vi "SLL DE Create DAQ INI File.vi"(8 "error in (no error)":errorcluster) -> (0 "error out":errorcluster)   [LabVIEW 2013]
doc: "Copyright © 2005, Soliton Technologies.\nAll rights reserved."
uses:
  Sub VIs/DAQ Engine/Controls/SLL DE List of Analog Outputs.ctl
  Sub VIs/DAQ Engine/Controls/SLL DE List of Digital Outputs.ctl
  Sub VIs/DAQ Engine/Controls/SLL DE DAQ Engine Parameters.ctl
  Sub VIs/DAQ Engine/Controls/SLL DE DAQ Parameters LV2Global Options.ctl
  Sub VIs/DAQ Engine/Controls/SLL DE List of Analog Inputs.ctl
  Sub VIs/DAQ Engine/Controls/SLL DE AO Min Max Range Checking Options.ctl
  Sub VIs/DAQ Engine/Controls/SLL DE List of AI Channel Type.ctl
panel:
  in  "DO Channel":T1=enum."STATION1_STOP TEST"
  in  "stop":bool
  in  "Tab Control":T2(tab)=enum."Page 11"
  in  "Stop":bool
  in  "Start":bool
  in  "Enable Acquisation and Control Types":T3={"Enable Analog Acqistation"=TRUE, "Enable Analog Control"=TRUE, "Enable Digital Acqistation"=TRUE, "Enable Digital Control"=TRUE}
  in  "OK 1":bool
  in  "DAQ Control Type":T4
  in  "OK 2":bool
  in  "DAQ Parameters":T5={"AI Sampling Rate (Samples/Sec)"=1000.0, "MvgAVG Window Size (# of Points)"=20, "Enable Filter"=TRUE, "Enable MvgAVG"=TRUE, "Circular Buffer Size (Sec)"=5.0, "AO Sampling Rate (Samples/Sec)"=1000.0, "Graph Update Rate (Samples/Sec)"=0.0, "File Logging Rate (Samples/Sec)"=500}
  in  "OK 3":bool
  in  "OK 4":bool
  in  "OK 5":bool
  in  "OK 6":bool
  in  "OK 7":bool
  in  "AO Safe Values":T7(array[cluster])
  in  "OK 8":bool
  in  "OK 9":bool
  in  "DO Safe Values":T8(array[cluster])
  in  "OK 10":bool
  in  "DO Interconnected Lines":T9(array[cluster])=[{"First DO Line"=enum."STATION1_STOP TEST", "Second DO Line"=enum."STATION1_START TEST"}]
  in  "OK 11":bool
  in  "AI Channels Unit":T12(array[cluster])
  in  "OK 12":bool
  in  "Units Information":T13(array[cluster])
  in  "Cancel?":bool
  in  "Write DAQ INI?":bool
  # "This is a automated DAQ INI File creation Vizard"
  # "Enable or disable the acquisation and control types and then Press OK"
  # "Populate AI"
  # "Populate AO"
  # "Populate DI"
  # "Populate DO"
  # "="
  # "-"
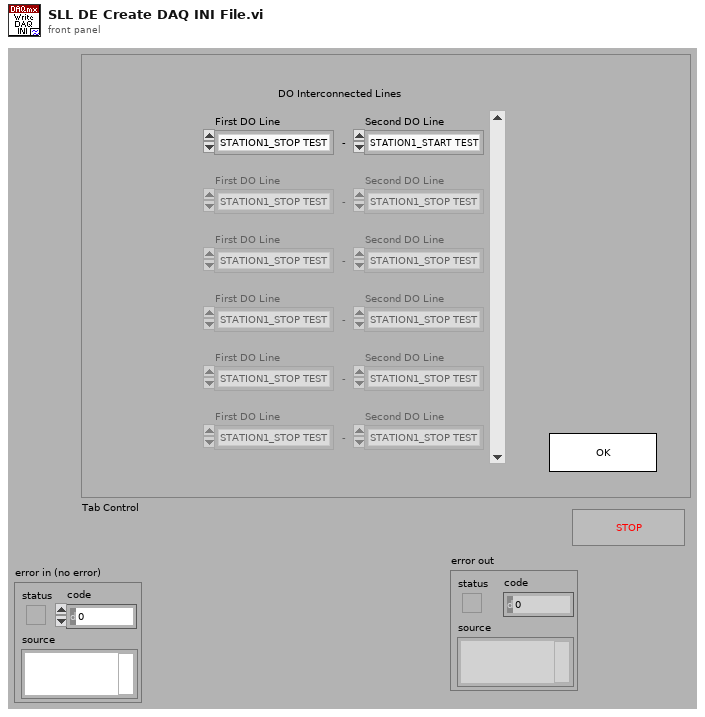
[diagram p1: front panel]
types:
  T1 = typedef "SLL DE List of Digital Outputs.ctl" = enum16{"STATION1_START TEST", "STATION1_STOP TEST", "STATION1_LIGHT1", "STATION1_LIGHT2", "STATION1_LIGHT3", "STATION1_SELECT_TEST", "STATION2_START TEST", "STATION2_STOP TEST", "STATION2_LIGHT1", "STATION2_LIGHT2", "STATION2_LIGHT3", "STATION2_SELECT_TEST", "STATION3_START TEST", "STATION3_STOP TEST", "STATION3_LIGHT1", "STATION3_LIGHT2", "STATION3_LIGHT3", "STATION3_SELECT_TEST", "STATION4_START TEST", "STATION4_STOP TEST", "STATION4_LIGHT1", "STATION4_LIGHT2", "STATION4_LIGHT3", "STATION4_SELECT_TEST"}
  T2 = enum32{"Page 1", "Page 2", "Page 3", "Page 4", "Page 5", "Page 6", "Page 7", "Page 8", "Page 9", "Page 10", "Page 11", "Page 12", "Page 13", "Page 14"}
  T3 = cluster{"Enable Analog Acqistation":bool, "Enable Analog Control":bool, "Enable Digital Acqistation":bool, "Enable Digital Control":bool}
  T4 = cluster{"Analog Input":enum16{"Finite", "Continuous", "Driver"}, "Analog Output":enum16{"Finite", "Continuous", "Driver"}, "Digital Input":enum16{"Finite", "Continuous", "Driver"}, "Digital Output":enum16{"Finite", "Continuous", "Driver"}}
  T5 = cluster{"AI Sampling Rate (Samples/Sec)":dbl, "MvgAVG Window Size (# of Points)":i32, "Enable Filter":bool, "Enable MvgAVG":bool, "Circular Buffer Size (Sec)":dbl, "AO Sampling Rate (Samples/Sec)":dbl, "Graph Update Rate (Samples/Sec)":dbl, "File Logging Rate (Samples/Sec)":i32}
  T6 = typedef "SLL DE List of Analog Outputs.ctl" = enum16{"None"}
  T7 = cluster{"Analog Outputs Name":T6, "Analog Outputs Safe Value":dbl}[]
  T8 = cluster{"Digital Outputs Name":T1, "Digital Outputs Safe Value":bool}[]
  T9 = cluster{"First DO Line":T1, "Second DO Line":T1}[]
  T10 = typedef "SLL DE List of Analog Inputs.ctl" = enum16{"None"}
  T11 = typedef "SLL DE List of AI Channel Type.ctl" = enum16{"Pressure", "Flow", "Temperature", "Time Scale", "Voltage", "Current", "Frequency", "Sound", "Speed", "Torque", "Distance", "Channel Type 1", "Channel Type 2", "Channel Type 3"}
  T12 = cluster{"Channel Name":T10, "Channel Type":T11}[]
  T13 = cluster{"Channel Type":T11, "Unit Text":string, "Maximum":dbl, "Minmum":dbl, "Increments":dbl}[]
  T14 = typedef "SLL DE DAQ Engine Parameters.ctl" = cluster{"Enable Engines":cluster{"AI Enable":bool, "AO Enable":bool, "DI Enable":bool, "DO Enable":bool}, "DAQ Control Type":cluster{"Analog Input":enum16{"Finite", "Continuous", "Driver"}, "Analog Output":enum16{"Finite", "Continuous", "Driver"}, "Digital Input":enum16{"Finite", "Continuous", "Driver"}, "Digital Output":enum16{"Finite", "Continuous", "Driver"}}, "DAQ Parameters":cluster{"AI Sampling Rate (Samples/Sec)":dbl, "MvgAVG Window Size (# of Points)":i32, "Enable Filter":bool, "Enable MvgAVG":bool, "Circular Buffer Size (Sec)":dbl, "AO Sampling Rate (Samples/Sec)":dbl, "Graph Update Rate (Samples/Sec)":dbl, "File Logging Rate (Samples/Sec)":i32}, "AO Safe Values":cluster{"Analog Outputs Name":T6, "Analog Outputs Safe Value":dbl}[], "DO Safe Values":cluster{"Digital Outputs Name":T1, "Digital Outputs Safe Value":bool}[], "DO Interconnected Lines":cluster{"First DO Line":string, "Second DO Line":string}[], "AI Channels Unit":cluster{"Channel Name":T10, "Channel Type":T11}[], "Units Information":cluster{"Channel Type":T11, "Unit Text":string, "Maximum":dbl, "Minmum":dbl, "Increments":dbl}[]}
  T15 = typedef "SLL DE AO Min Max Range Checking Options.ctl" = enum16{"Initalize Channel Range", "Check Single AO Channel", "Check Multiple AO Channels"}
  T16 = typedef "SLL DE DAQ Parameters LV2Global Options.ctl" = enum16{"Read", "Write"}
  T17 = cluster{"List of Analog Outputs":T6, "value":dbl}
  T18 = cluster{"List of Digital Outputs":T1, "value":bool}
  T19 = cluster{"AI Enable":bool, "AO Enable":bool, "DI Enable":bool, "DO Enable":bool}
  T20 = cluster{"List of Analog Inputs":T10, "Channel Type":T11}[]
  T21 = cluster{"List of Digital Outputs":T1, "List of Digital Outputs":T1}
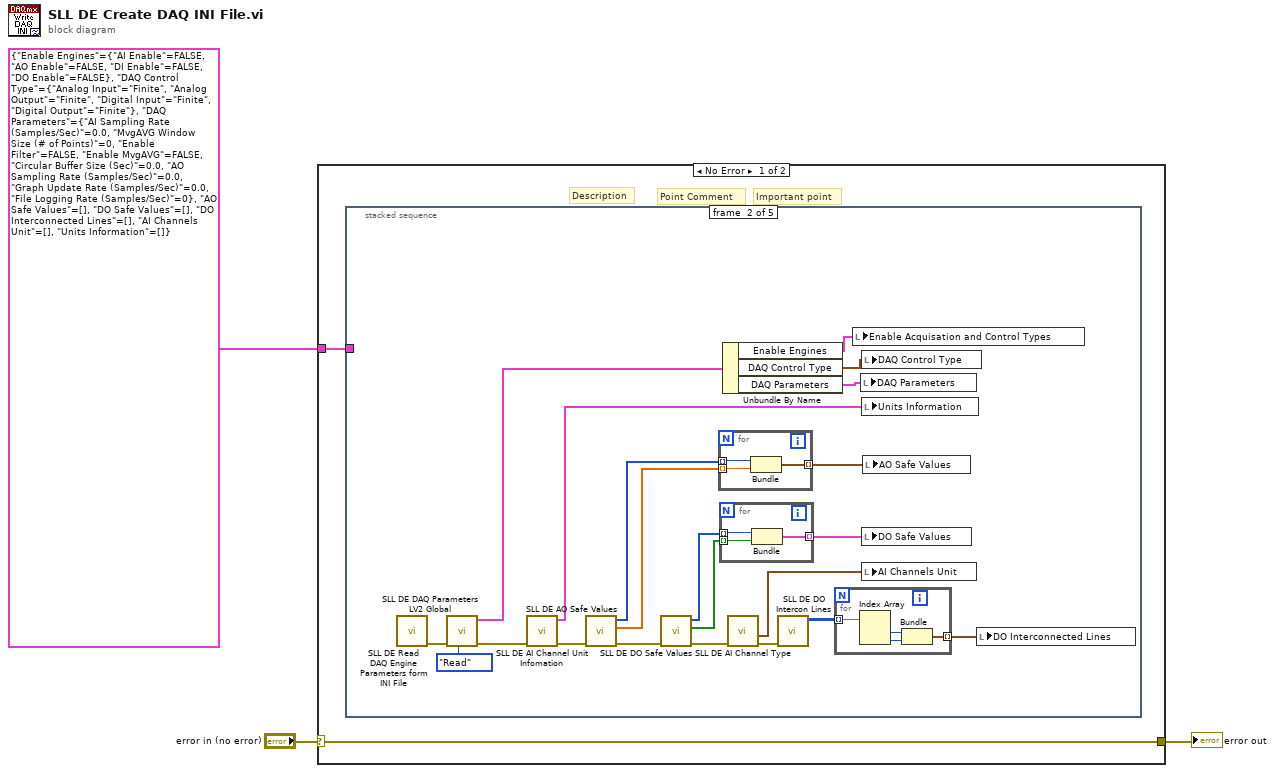
[diagram p0: block diagram]
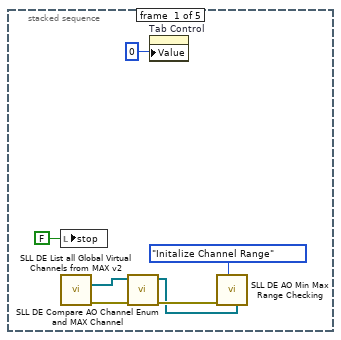
[diagram p2: hidden frame]
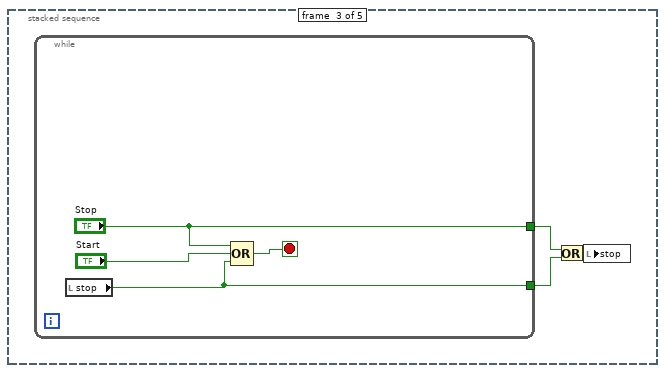
[diagram p3: hidden frame]
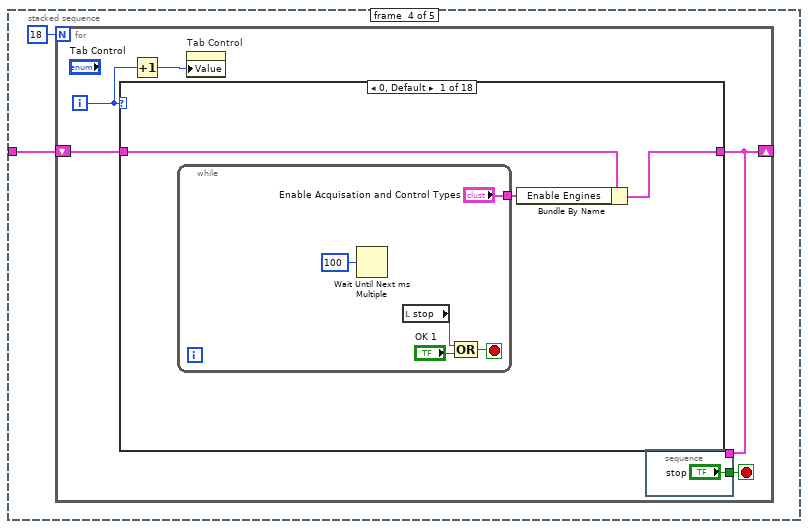
[diagram p4: hidden frame]
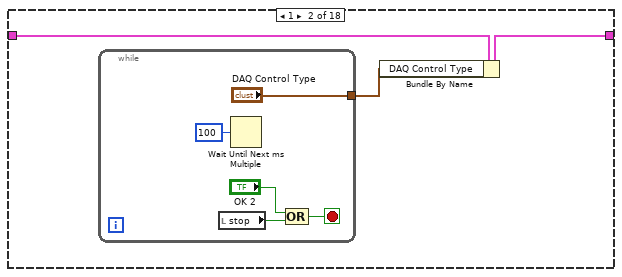
[diagram p5: hidden frame]
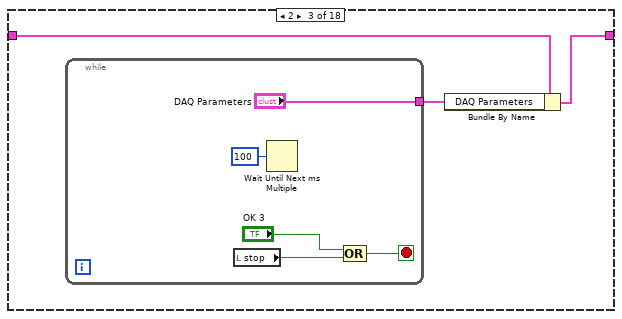
[diagram p6: hidden frame]
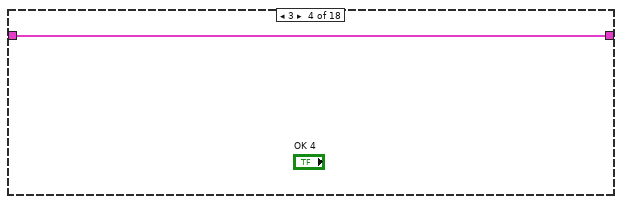
[diagram p7: hidden frame]
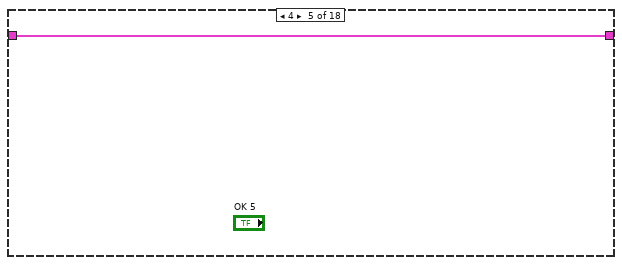
[diagram p8: hidden frame]
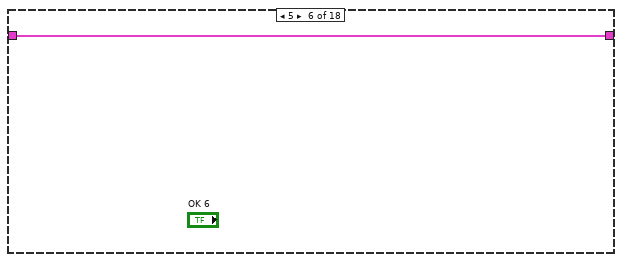
[diagram p9: hidden frame]
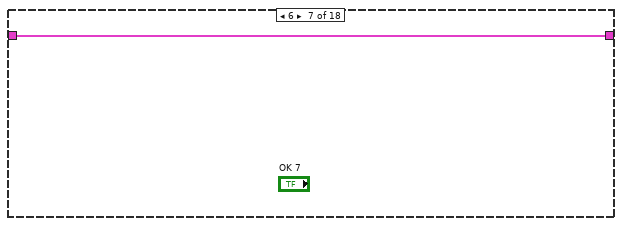
[diagram p10: hidden frame]
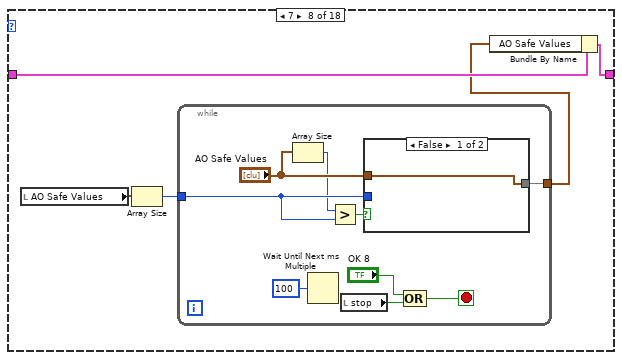
[diagram p11: hidden frame]
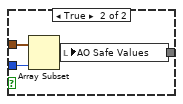
[diagram p12: hidden frame]
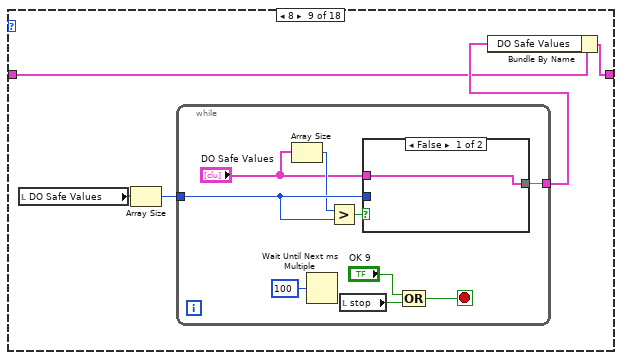
[diagram p13: hidden frame]
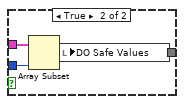
[diagram p14: hidden frame]
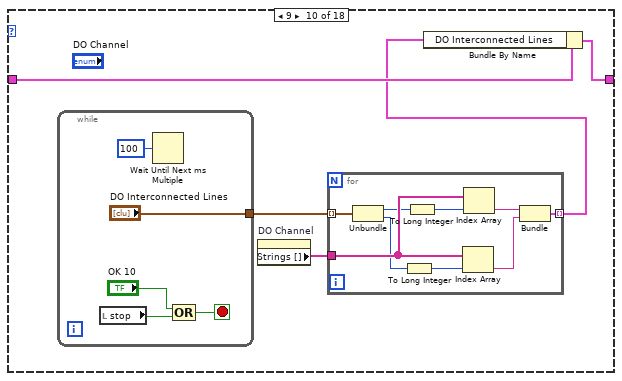
[diagram p15: hidden frame]
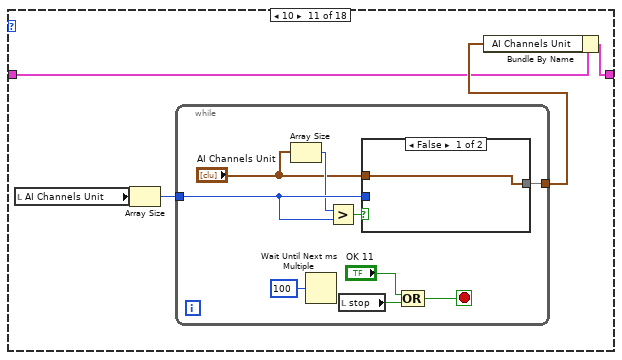
[diagram p16: hidden frame]
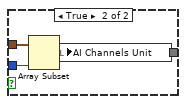
[diagram p17: hidden frame]
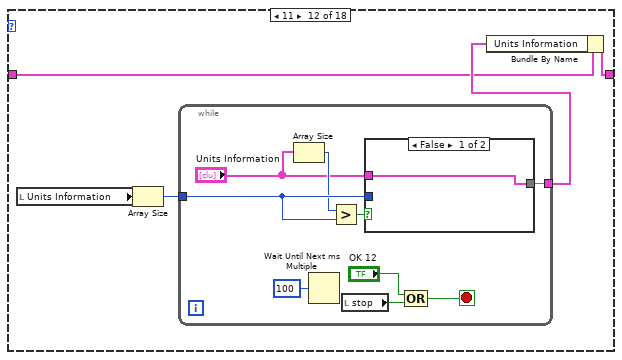
[diagram p18: hidden frame]
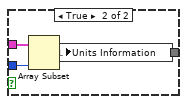
[diagram p19: hidden frame]
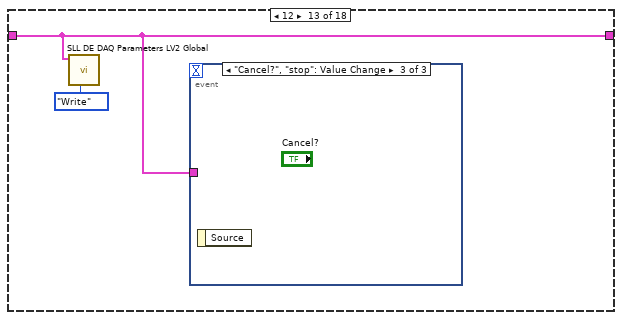
[diagram p20: hidden frame]
diagram:
  n1 = case shown="No Error" "error in (no error)" {
    selector: "error in (no error)" -> [w5 w189]
    tunnel: [w5 w189] -> w2
    tunnel: T14 {"Enable Engines"={"AI Enable"=FALSE, "AO Enable"=FALSE, "DI Enable"=FALSE, "DO Enable"=FALSE}, "DAQ Control Type"={"Analog Input"=enum."Finite", "Analog Output"=enum."Finite", "Digital Input"=enum."Finite", "Digital Output"=enum."Finite"}, "DAQ Parameters"={"AI Sampling Rate (Samples/Sec)"=0.0, "MvgAVG Window Size (# of Points)"=0, "Enable Filter"=FALSE, "Enable MvgAVG"=FALSE, "Circular Buffer Size (Sec)"=0.0, "AO Sampling Rate (Samples/Sec)"=0.0, "Graph Update Rate (Samples/Sec)"=0.0, "File Logging Rate (Samples/Sec)"=0}, "AO Safe Values"=[], "DO Safe Values"=[], "DO Interconnected Lines"=[], "AI Channels Unit"=[], "Units Information"=[]} ("DAQ Engine") -> [w4 _]
    frame No Error {
      # "Point Comment"
      # "Important point"
      # "Description"
      n2 = stacked-sequence {
        tunnel: w4 -> [_ _ _ w51 _]
        frame #0 {
          n3 = local write "stop"(FALSE ("stop")) -> ()
          n4 = call "SLL DE List all Global Virtual Channels from MAX v2.vi"() -> ("error out"=w8:errorcluster, "Analog Output"=w10:refnum<k21>[])  [unwired: 5 in, 5 out]
          n5 = call "SLL DE Compare AO Channel Enum and MAX Channel.vi"("error in (no error)"=w8, "Analog Output Channels"=w10) -> ("error out"=w9:errorcluster, "Channels Out"=w7:refnum<k21>[])  [unwired: 7 in, 1 out]
          n6 = property on="Tab Control" class="TabCtl (strict)"("Value"=0) -> ()  [unwired: 2 in, 2 out]
          n7 = call "SLL DE AO Min Max Range Checking.vi"("Analog Output Channels"=w7, "Option"=SLL_DE_AO_Min_Max_Range_Checking_Options."Initalize Channel Range", "error in (no error)"=w9) -> ()  [unwired: 6 in, 3 out]
        }
        frame #1 {
          n8 = call "SLL DE Read DAQ Engine Parameters form INI File.vi"() -> ("error out"=w32:errorcluster)  [unwired: 11 in]
          n9 = call "SLL DE DAQ Parameters LV2 Global.vi"("Option"=SLL_DE_DAQ_Parameters_LV2Global_Options."Read", "Error in (no error)"=w32) -> ("Error out"=w15:errorcluster, "Global Info"=w31:T14)  [unwired: 8 in]
          n10 = call "SLL DE AI Channel Unit Infomation.vi"("error in (no error)"=w15) -> ("error out"=w14:errorcluster, "Unit Infomation"=w13:T13)  [unwired: 9 in]
          n11 = call "SLL DE AO Safe Values.vi"("error in (no error)"=w14) -> ("error out"=w22:errorcluster, "AO Safe Values"=w24:dbl[], "AO Channels (Enum)"=w25:T6[])  [unwired: 8 in]
          n12 = call "SLL DE DO Safe Values.vi"("error in (no error)"=w22) -> ("error out"=w17:errorcluster, "DO Safe Values"=w20:bool[], "DO Name"=w21:T1[])  [unwired: 8 in]
          n13 = for {
            tunnel: w25 -> [w39] mode=indexing
            tunnel: w24 -> [w38] mode=indexing
            tunnel: [w37] -> w23 mode=indexing
            n14 = Bundle("List of Analog Outputs"=w39, "value"=w38) -> (w37:T17)  [unwired: 1 in]
          }
          n15 = for {
            tunnel: w21 -> [w36] mode=indexing
            tunnel: w20 -> [w35] mode=indexing
            tunnel: [w34] -> w19 mode=indexing
            n16 = Bundle("List of Digital Outputs"=w36, "value"=w35) -> (w34:T18)  [unwired: 1 in]
          }
          n17 = Unbundle By Name(w31) -> ("Enable Engines"=w30:T19, "DAQ Control Type"=w29:T4, "DAQ Parameters"=w28:T5)
          n18 = call "SLL DE AI Channel Type.vi"("error in (no error)"=w17) -> ("error out"=w16:errorcluster, "AI Channels Unit"=w18:T20)  [unwired: 7 in, 2 out]
          n19 = call "SLL DE DO Intercon Lines.vi"("Error In"=w16) -> ("DO Name"=w27:T1[][])  [unwired: 9 in, 1 out]
          n20 = for {
            tunnel: w27 -> [w43] mode=indexing
            tunnel: [w40] -> w26 mode=indexing
            n21 = Index Array(array=w43) -> (element #1=w42:T1, element #2=w41:T1)  [unwired: 2 in]
            n22 = Bundle("List of Digital Outputs"=w42, "List of Digital Outputs"=w41) -> (w40:T21)  [unwired: 1 in]
          }
          n23 = local write "Enable Acquisation and Control Types"(w30) -> ()
          n24 = local write "DAQ Parameters"(w28) -> ()
          n25 = local write "DAQ Control Type"(w29) -> ()
          n26 = local write "Units Information"(w13) -> ()
          n27 = local write "DO Safe Values"(w19) -> ()
          n28 = local write "AI Channels Unit"(w18) -> ()
          n29 = local write "AO Safe Values"(w23) -> ()
          n30 = local write "DO Interconnected Lines"(w26) -> ()
        }
        frame #2 {
          n31 = while {
            tunnel: ["Stop"] -> w45
            tunnel: [w47] -> w44
            stop <- w49 stop-if-true
            n32 = local read "stop"() -> (w47:bool)
            n33 = Compound Arithmetic op=OR("Stop", "Start", w47) -> (w49:bool)
          }
          n34 = Or(x=w45, y=w44) -> (x .or. y?=w46:bool)
          n35 = local write "stop"(w46) -> ()
        }
        frame #3 {
          n36 = for {
            N: 18 -> [_]
            shift-right: [w53] -> _
            shift-left: w51 -> [w57]
            i -> [w55]
            stop <- w54 stop-if-true
            n37 = case shown="0, Default" w55 {
              tunnel: w57 -> [w61 w69 w77 w83 w84 w85 w86 w91 w106 w127 w143 w161 w178 w183 w184 w185 w186 w187]
              tunnel: [w60 w68 w76 w83 w84 w85 w86 w90 w105 w126 w142 w160 w178 w183 w184 w185 w186 w187] -> w53
              frame 0, Default {
                n38 = while {
                  tunnel: ["Enable Acquisation and Control Types"] -> w59
                  stop <- w63 stop-if-true
                  n39 = Wait Until Next ms Multiple(millisecond multiple=u32 100) -> ()  [unwired: 1 out]
                  n40 = local read "stop"() -> (w62:bool)
                  n41 = Compound Arithmetic op=OR(w62, "OK 1") -> (w63:bool)
                }
                n42 = Bundle By Name(cluster=w61, "Enable Engines"=w59) -> (w60:T14)
              }
              frame 1 {
                n43 = while {
                  tunnel: ["DAQ Control Type"] -> w67
                  stop <- w72 stop-if-true
                  n44 = local read "stop"() -> (w71:bool)
                  n45 = Wait Until Next ms Multiple(millisecond multiple=u32 100) -> ()  [unwired: 1 out]
                  n46 = Compound Arithmetic op=OR("OK 2", w71) -> (w72:bool)
                }
                n47 = Bundle By Name(cluster=w69, "DAQ Control Type"=w67) -> (w68:T14)
              }
              frame 2 {
                n48 = while {
                  tunnel: ["DAQ Parameters"] -> w75
                  stop <- w80 stop-if-true
                  n49 = local read "stop"() -> (w81:bool)
                  n50 = Wait Until Next ms Multiple(millisecond multiple=u32 100) -> ()  [unwired: 1 out]
                  n51 = Compound Arithmetic op=OR("OK 3", w81) -> (w80:bool)
                }
                n52 = Bundle By Name(cluster=w77, "DAQ Parameters"=w75) -> (w76:T14)
              }
              frame 3 {
              }
              frame 4 {
              }
              frame 5 {
              }
              frame 6 {
              }
              frame 7 {
                n53 = local read "AO Safe Values"() -> (w88:T7)
                n54 = Array Size(array=w88) -> (size(s)=w87:i32)
                n55 = while {
                  tunnel: [w94] -> w89
                  tunnel: w87 -> [w95]
                  stop <- w99 stop-if-true
                  n56 = Array Size(array="AO Safe Values") -> (size(s)=w93:i32)
                  n57 = Wait Until Next ms Multiple(millisecond multiple=u32 100) -> ()  [unwired: 1 out]
                  n58 = Greater?(x=w93, y=w95) -> (0:w92:bool)
                  n59 = local read "stop"() -> (w100:bool)
                  n60 = case shown="False" w92 {
                    tunnel: w95 -> [_ w104]
                    tunnel: "AO Safe Values" -> [w101 w103]
                    tunnel: [w101 w102] -> w94
                    frame False {
                    }
                    frame True {
                      n61 = Array Subset(array=w103, length=w104) -> (w102:T7)  [unwired: 1 in]
                      n62 = local write "AO Safe Values"(w102) -> ()
                    }
                  }
                  n63 = Compound Arithmetic op=OR("OK 8", w100) -> (w99:bool)
                }
                n64 = Bundle By Name(cluster=w91, "AO Safe Values"=w89) -> (w90:T14)
              }
              frame 8 {
                n65 = local read "DO Safe Values"() -> (w108:T8)
                n66 = Array Size(array=w108) -> (size(s)=w107:i32)
                n67 = while {
                  tunnel: [w114] -> w109
                  tunnel: w107 -> [w115]
                  stop <- w117 stop-if-true
                  n68 = Array Size(array="DO Safe Values") -> (size(s)=w113:i32)
                  n69 = Wait Until Next ms Multiple(millisecond multiple=u32 100) -> ()  [unwired: 1 out]
                  n70 = Greater?(x=w113, y=w115) -> (0:w112:bool)
                  n71 = local read "stop"() -> (w118:bool)
                  n72 = case shown="False" w112 {
                    tunnel: w115 -> [_ w122]
                    tunnel: "DO Safe Values" -> [w119 w121]
                    tunnel: [w119 w120] -> w114
                    frame False {
                    }
                    frame True {
                      n73 = Array Subset(array=w121, length=w122) -> (w120:T8)  [unwired: 1 in]
                      n74 = local write "DO Safe Values"(w120) -> ()
                    }
                  }
                  n75 = Compound Arithmetic op=OR("OK 9", w118) -> (w117:bool)
                }
                n76 = Bundle By Name(cluster=w106, "DO Safe Values"=w109) -> (w105:T14)
              }
              frame 9 {
                n77 = while {
                  tunnel: ["DO Interconnected Lines"] -> w125
                  stop <- w139 stop-if-true
                  n78 = local read "stop"() -> (w141:bool)
                  n79 = Wait Until Next ms Multiple(millisecond multiple=u32 100) -> ()  [unwired: 1 out]
                  n80 = Compound Arithmetic op=OR("OK 10", w141) -> (w139:bool)
                }
                n81 = property on="DO Channel" class="Enum (strict)"() -> ("Strings []"=w124:string[])  [unwired: 2 in, 2 out]
                n82 = for {
                  tunnel: w125 -> [w136] mode=indexing
                  tunnel: w124 -> [w135]
                  tunnel: [w128] -> w123 mode=indexing
                  n83 = Unbundle(w136) -> ("First DO Line"=w134:T1, "Second DO Line"=w133:T1)
                  n84 = To Long Integer(number=w133) -> (32bit integer=w131:i32)
                  n85 = To Long Integer(number=w134) -> (32bit integer=w132:i32)
                  n86 = Index Array(array=w135, index=w131) -> (element=w129:string)
                  n87 = Index Array(array=w135, index=w132) -> (element=w130:string)
                  n88 = Bundle(w130, w129) -> (w128:cluster{string, string})  [unwired: 1 in]
                }
                n89 = Bundle By Name(cluster=w127, "DO Interconnected Lines"=w123) -> (w126:T14)
              }
              frame 10 {
                n90 = local read "AI Channels Unit"() -> (w145:T12)
                n91 = Array Size(array=w145) -> (size(s)=w144:i32)
                n92 = while {
                  tunnel: [w151] -> w146
                  tunnel: w144 -> [w152]
                  stop <- w154 stop-if-true
                  n93 = Array Size(array="AI Channels Unit") -> (size(s)=w150:i32)
                  n94 = Wait Until Next ms Multiple(millisecond multiple=u32 100) -> ()  [unwired: 1 out]
                  n95 = Greater?(x=w150, y=w152) -> (0:w149:bool)
                  n96 = local read "stop"() -> (w155:bool)
                  n97 = case shown="False" w149 {
                    tunnel: w152 -> [_ w159]
                    tunnel: "AI Channels Unit" -> [w156 w158]
                    tunnel: [w156 w157] -> w151
                    frame False {
                    }
                    frame True {
                      n98 = Array Subset(array=w158, length=w159) -> (w157:T12)  [unwired: 1 in]
                      n99 = local write "AI Channels Unit"(w157) -> ()
                    }
                  }
                  n100 = Compound Arithmetic op=OR("OK 11", w155) -> (w154:bool)
                }
                n101 = Bundle By Name(cluster=w143, "AI Channels Unit"=w146) -> (w142:T14)
              }
              frame 11 {
                n102 = local read "Units Information"() -> (w163:T13)
                n103 = Array Size(array=w163) -> (size(s)=w162:i32)
                n104 = while {
                  tunnel: [w169] -> w164
                  tunnel: w162 -> [w170]
                  stop <- w172 stop-if-true
                  n105 = Array Size(array="Units Information") -> (size(s)=w168:i32)
                  n106 = Wait Until Next ms Multiple(millisecond multiple=u32 100) -> ()  [unwired: 1 out]
                  n107 = Greater?(x=w168, y=w170) -> (0:w167:bool)
                  n108 = local read "stop"() -> (w173:bool)
                  n109 = case shown="False" w167 {
                    tunnel: w170 -> [_ w177]
                    tunnel: "Units Information" -> [w174 w176]
                    tunnel: [w174 w175] -> w169
                    frame False {
                    }
                    frame True {
                      n110 = Array Subset(array=w176, length=w177) -> (w175:T13)  [unwired: 1 in]
                      n111 = local write "Units Information"(w175) -> ()
                    }
                  }
                  n112 = Compound Arithmetic op=OR("OK 12", w173) -> (w172:bool)
                }
                n113 = Bundle By Name(cluster=w161, "Units Information"=w164) -> (w160:T14)
              }
              frame 12 {
                n114 = call "SLL DE DAQ Parameters LV2 Global.vi"("Option"=SLL_DE_DAQ_Parameters_LV2Global_Options."Write", "Global Info"=w178) -> ()  [unwired: 8 in, 2 out]
                n115 = event shown="[2] \"Cancel?\", \"stop\": Value Change" {
                  selector: _ -> [_ _ _]
                  dyn-events: _ -> [_ _ _]
                  timeout: _ -> [_ _ _]
                  tunnel: w178 -> [_ w181 _]
                  event Timeout {
                    n116 = event-data() -> ()  [unwired: 1 in, 2 out]
                  }
                  event "Write DAQ INI?": Value Change {
                    n117 = event-data() -> ()  [unwired: 1 in, 1 out]
                    n118 = call "SLL DE DAQ Parameters LV2 Global.vi"("Option"=SLL_DE_DAQ_Parameters_LV2Global_Options."Write", "Global Info"=w181) -> ("Error out"=w180:errorcluster)  [unwired: 8 in, 1 out]
                    n119 = call "SLL DE Write DAQ Engine Parameters form INI File.vi"("error in (no error)"=w180) -> ()  [unwired: 10 in, 1 out]
                  }
                  event "Cancel?", "stop": Value Change {
                    n120 = event-data() -> ()  [unwired: 1 in, 1 out]
                  }
                }
              }
              frame 13 {
              }
              frame 14 {
              }
              frame 15 {
              }
              frame 16 {
              }
              frame 17 {
              }
            }
            n121 = Increment(x=w55) -> (x+1=w56:i32)
            n122 = property on="Tab Control" class="TabCtl (strict)"("Value"=w56) -> ()  [unwired: 2 in, 2 out]
            n123 = stacked-sequence {
              tunnel: ["stop"] -> w54
              tunnel: w53 -> [_]
              frame #0 {
              }
            }
          }
        }
        frame #4 {
          n124 = local write "stop"(FALSE ("stop")) -> ()
        }
      }
    }
    frame Error {
    }
  }
  "error out" <- w2
